vi "测试.vi"() -> ()   [LabVIEW 2018]
panel:
  in  "数值":dbl
  in  "停止":bool
  out "Output Value":dbl format="%.2f"
  out "系统通讯故障":bool
  out "系统通讯正常":bool
  out "loadapp":i32 caption="port copy"
  out "tcpip":i32 caption="Port"
  in  "IP Port":string="22222"
  in  "IP Address":string="192.168.0.10"
  in  "Application filename":string="aa"
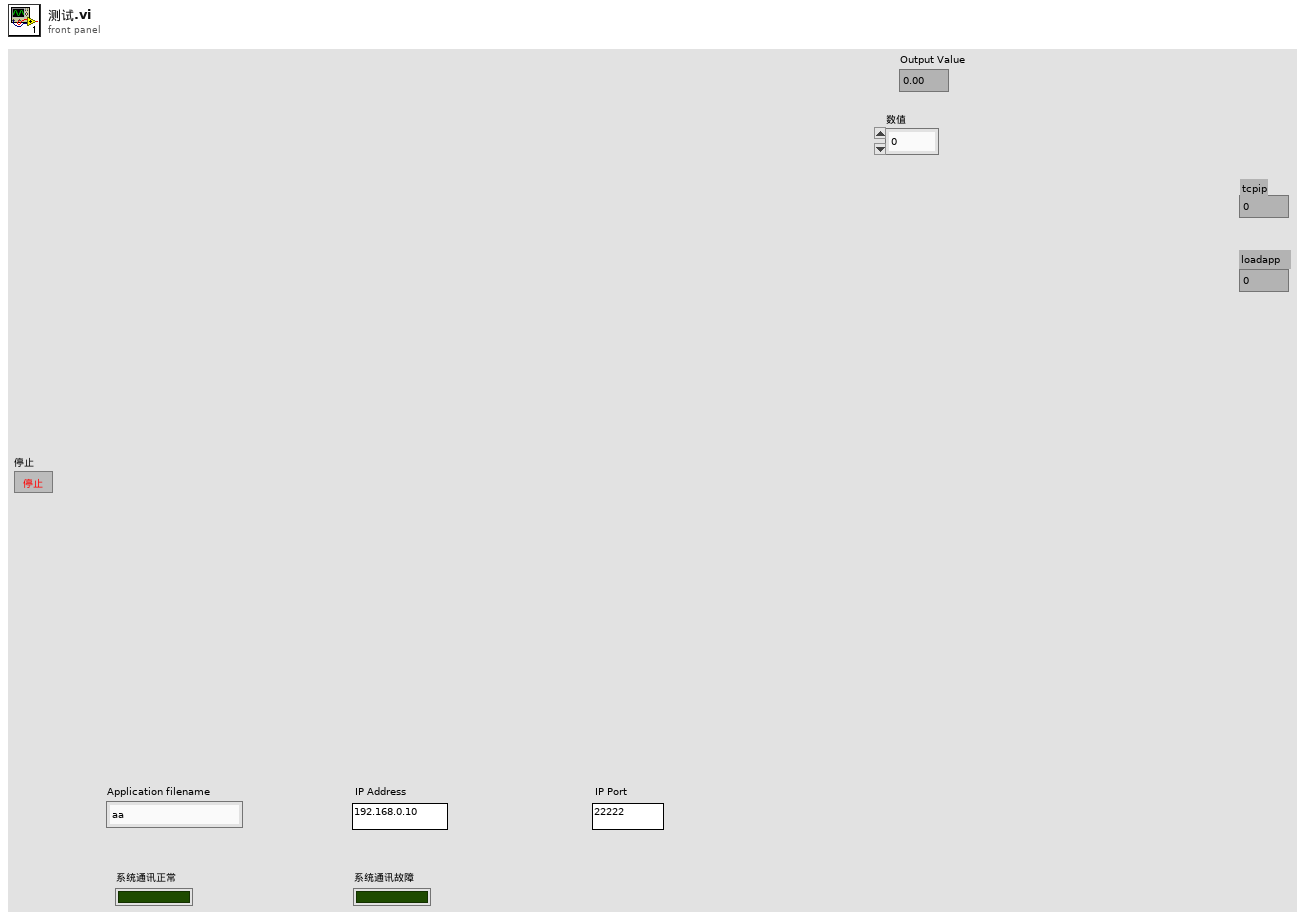
[diagram p1: front panel]
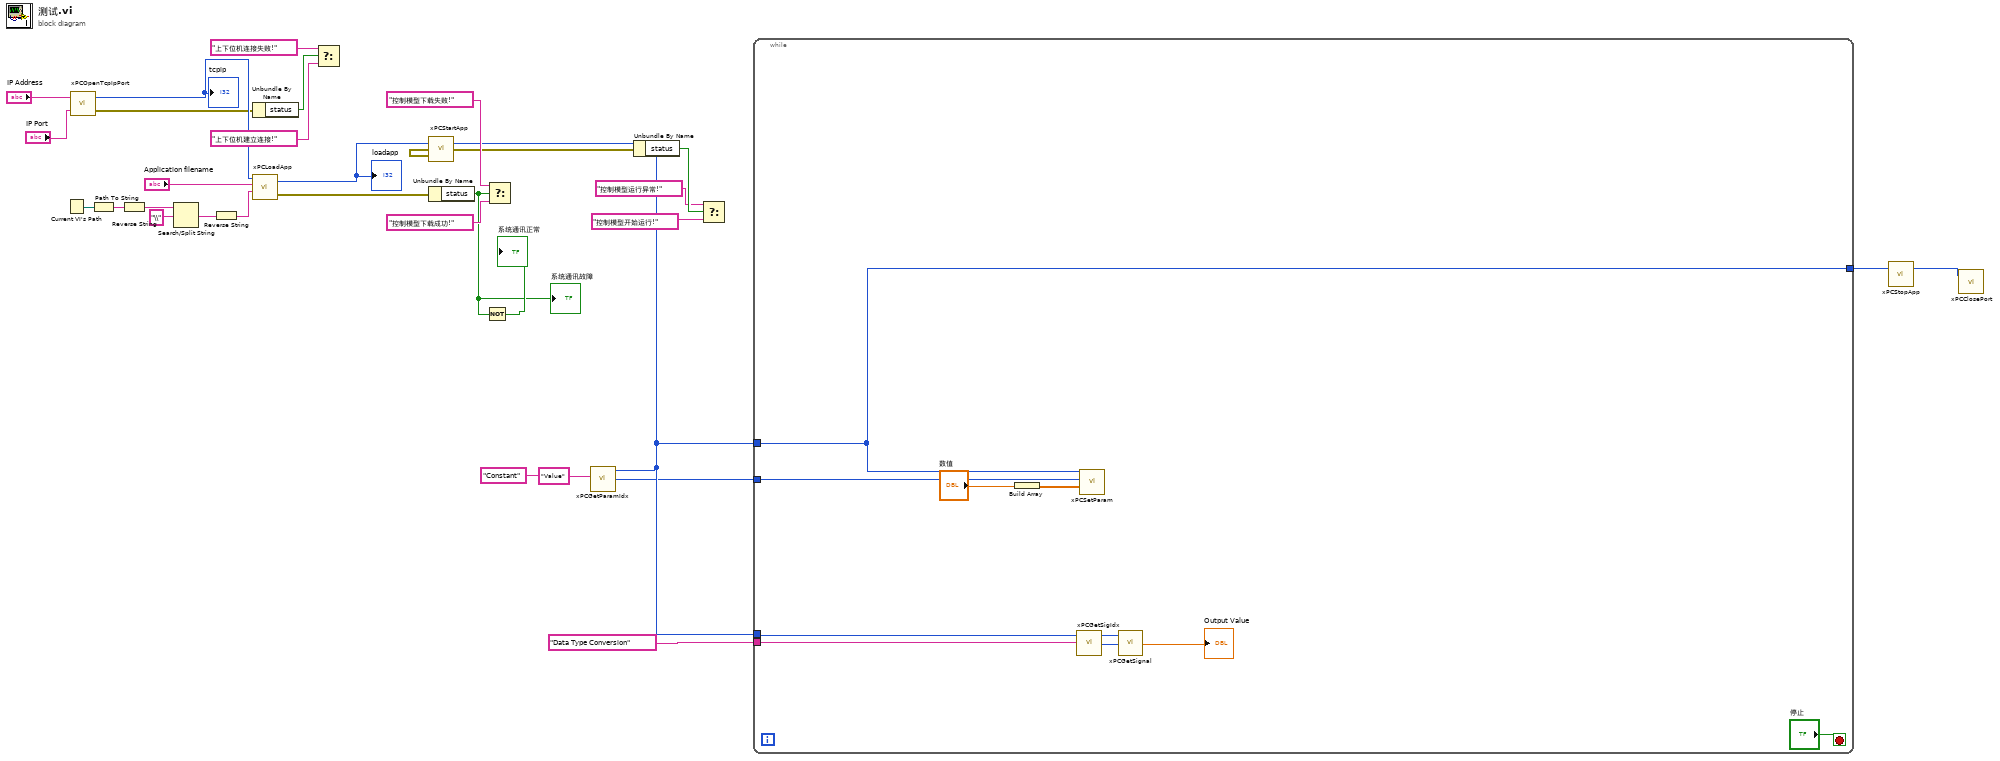
[diagram p0: block diagram]
diagram:
  n1 = Current VI's Path() -> (path=w25:path)
  n2 = call "xPCOpenTcpIpPort.vi"("port"="IP Port", "address"="IP Address") -> ("error out"=w16:errorcluster, "Port"=w17:i32)
  "tcpip" <- w17
  n3 = Path To String(path=w25) -> (string=w27:string)
  n4 = Reverse String(1:w27) -> (0:w29:string)
  n5 = Search/Split String(string=w29, search string/char (-)="\\" ("search char (-)")) -> (match + rest of string=w28:string)  [unwired: 1 in, 2 out]
  n6 = Reverse String(1:w28) -> (0:w30:string)
  n7 = Unbundle By Name(w16) -> ("status"=w23:bool)
  n8 = call "xPCLoadApp.vi"("pathstr"=w30, "filename"="Application filename", "port"=w17) -> ("error out"=w18:errorcluster, "port copy"=w24:i32)  [unwired: 1 in]
  "loadapp" <- w24
  n9 = Select(t="上下位机连接失败!" ("message"), s=w23, f="上下位机建立连接!" ("message")) -> ()  [unwired: 1 out]
  n10 = call "xPCStartApp.vi"("port"=w24) -> ("error out"=w10:errorcluster, "port copy"=w4:i32)  [unwired: 1 in]
  n11 = Unbundle By Name(w18) -> ("status"=w8:bool)
  "系统通讯故障" <- w8
  n12 = Not(x=w8) -> (.not. x?=→"系统通讯正常":bool)
  n13 = Select(t="控制模型下载失败!" ("message"), s=w8, f="控制模型下载成功!" ("message")) -> ()  [unwired: 1 out]
  n14 = call "xPCGetParamIdx.vi"("blockpath"="Constant" ("pathstr"), "parametername"="Value" ("filename"), "port"=w4) -> ("identifier"=w3:i32)  [unwired: 1 in, 2 out]
  n15 = Unbundle By Name(w10) -> ("status"=w12:bool)
  n16 = Select(t="控制模型运行异常!" ("message"), s=w12, f="控制模型开始运行!" ("message")) -> ()  [unwired: 1 out]
  n17 = while {
    tunnel: "Data Type Conversion" ("pathstr") -> [w39]
    tunnel: w4 -> [w38]
    tunnel: w4 -> [w32]
    tunnel: w3 -> [w35]
    tunnel: [w32] -> w1
    stop <- "停止" stop-if-true
    n18 = Build Array("数值") -> (w33:dbl[])
    n19 = call "xPCGetSigIdx.vi"("blockpath"=w39, "port"=w38) -> ("identifier"=w40:i32, "port copy"=w41:i32)  [unwired: 1 in, 1 out]
    n20 = call "xPCSetParam.vi"("value"=w33, "index"=w35, "port"=w32) -> ()  [unwired: 1 in, 2 out]
    n21 = call "xPCGetSignal.vi"("signal"=w40, "port"=w41) -> ("Output Value"=→"Output Value":dbl)  [unwired: 1 in, 2 out]
  }
  n22 = call "xPCStopApp.vi"("port"=w1) -> ("port copy"=w2:i32)  [unwired: 1 in, 1 out]
  n23 = call "xPCClosePort.vi"("port"=w2) -> ()  [unwired: 1 in, 2 out]
